vi "Yokogawa_original.vi"() -> ()   [LabVIEW 2020]
uses:
  <instrlib>/Yokogawa GX Series/Public/Data/Read Measurement Data (Analog NChan).vi
  <instrlib>/Yokogawa GX Series/Yokogawa GX Series.lvlib
panel:
  in  "prerun period":dbl=60.0
  in  "Serial Configuration":T1={"Baud Rate"=9600, "Parity"=2, "Data Bits"=8, "Flow Control"=0} {"Flow Control" items=["None", "XON/XOFF", "RTS/CTS", "XON/XOFF & RTS/CTS"]; "Data Bits" items=["7"=7, "8"=8]; "Parity" items=["None", "Odd", "Even"]; "Baud Rate" items=["1200"=1200, "2400"=2400, "4800"=4800, "9600"=9600, "19200"=19200, "38400"=38400, "57600"=57600, "115200"=115200]}
  in  "Specified\nTemperature\nLimit":dbl
  out "Time in Seconds":dbl
  out "String":string
  in  "Stop":bool
  out "Current":dbl
  out "Waveform Chart":dbl[][](graph)
  out "Current Data":dbl[](array[numeric])
  out "Unit":string[](array[string])
  out "Channel":string[](array[string])
  out "Time Stamp":timestamp
  in  "End Channel":string="0102"
  in  "Start Channel":string="0001"
  in  "VISA resource name":refnum<visa-resource-name>
  in  "Interval":dbl=5000.0
  # "Data \nacquisition \nfrequency\n(ms)"
  # "0001"
  # "0010 default \nor however many channels you want"
  # "60"
  # "Device IP On VI Max"
  # "9600"
  # "2"
  # "8"
  # "0"
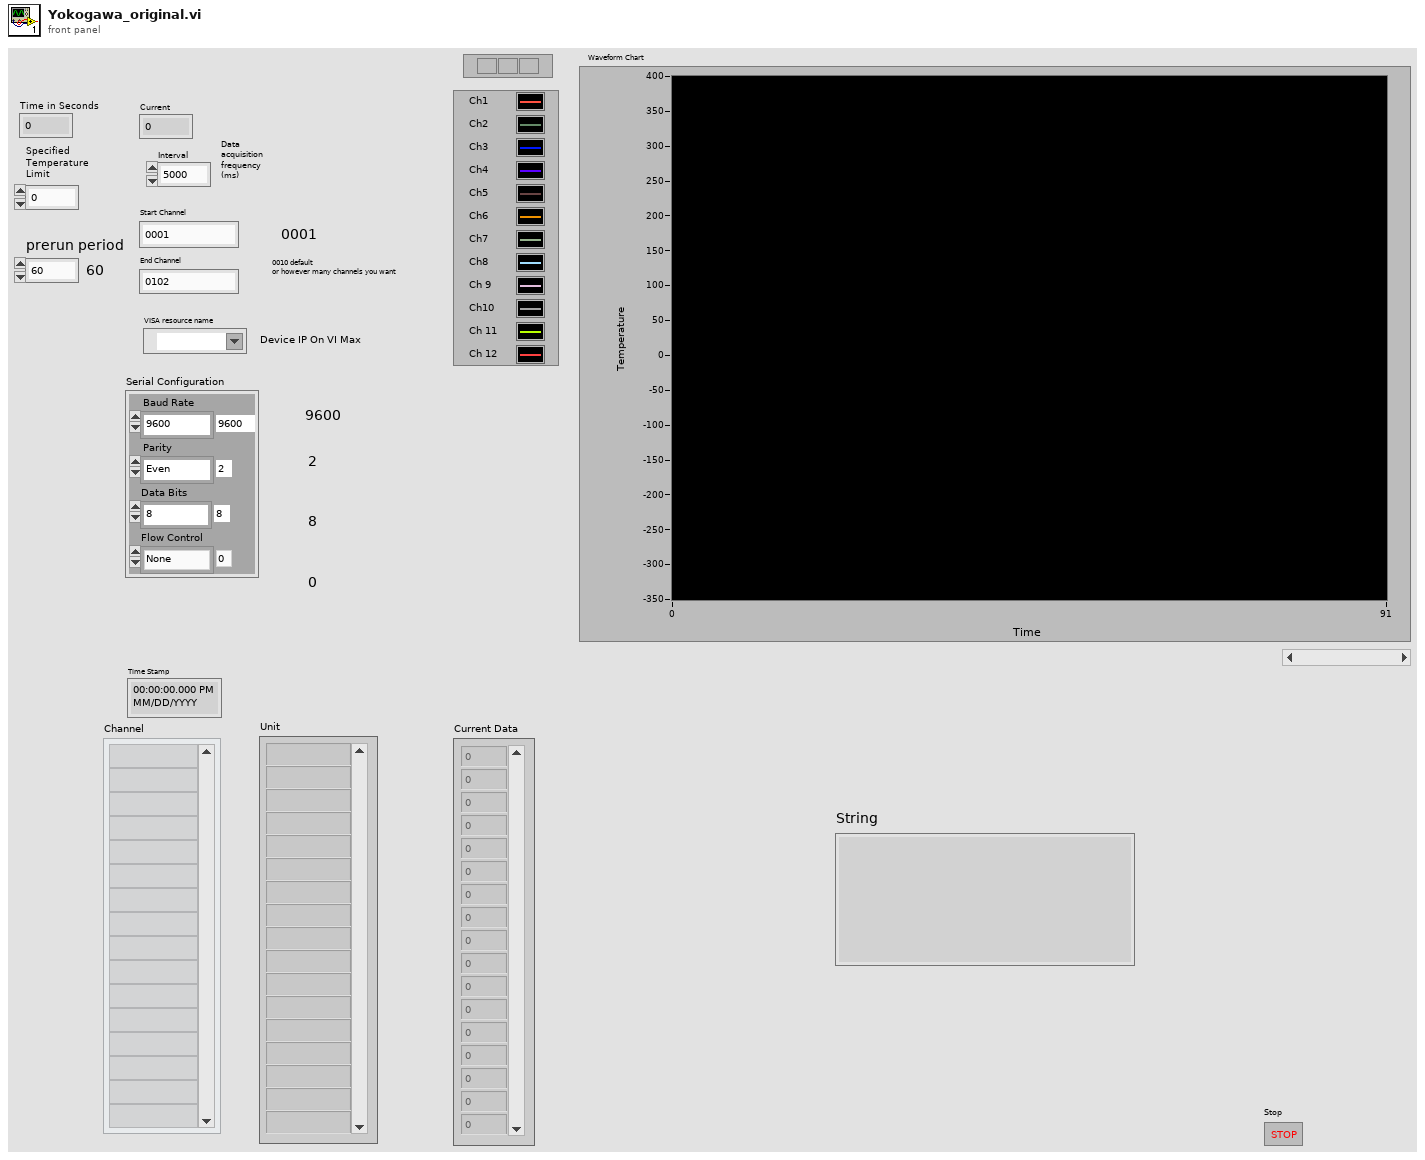
[diagram p1: front panel]
types:
  T1 = cluster{"Baud Rate":u32, "Parity":u16, "Data Bits":u16, "Flow Control":u16}
  T2 = enum16{"open", "replace", "create", "open or create", "replace or create", "replace or create with confirmation"}
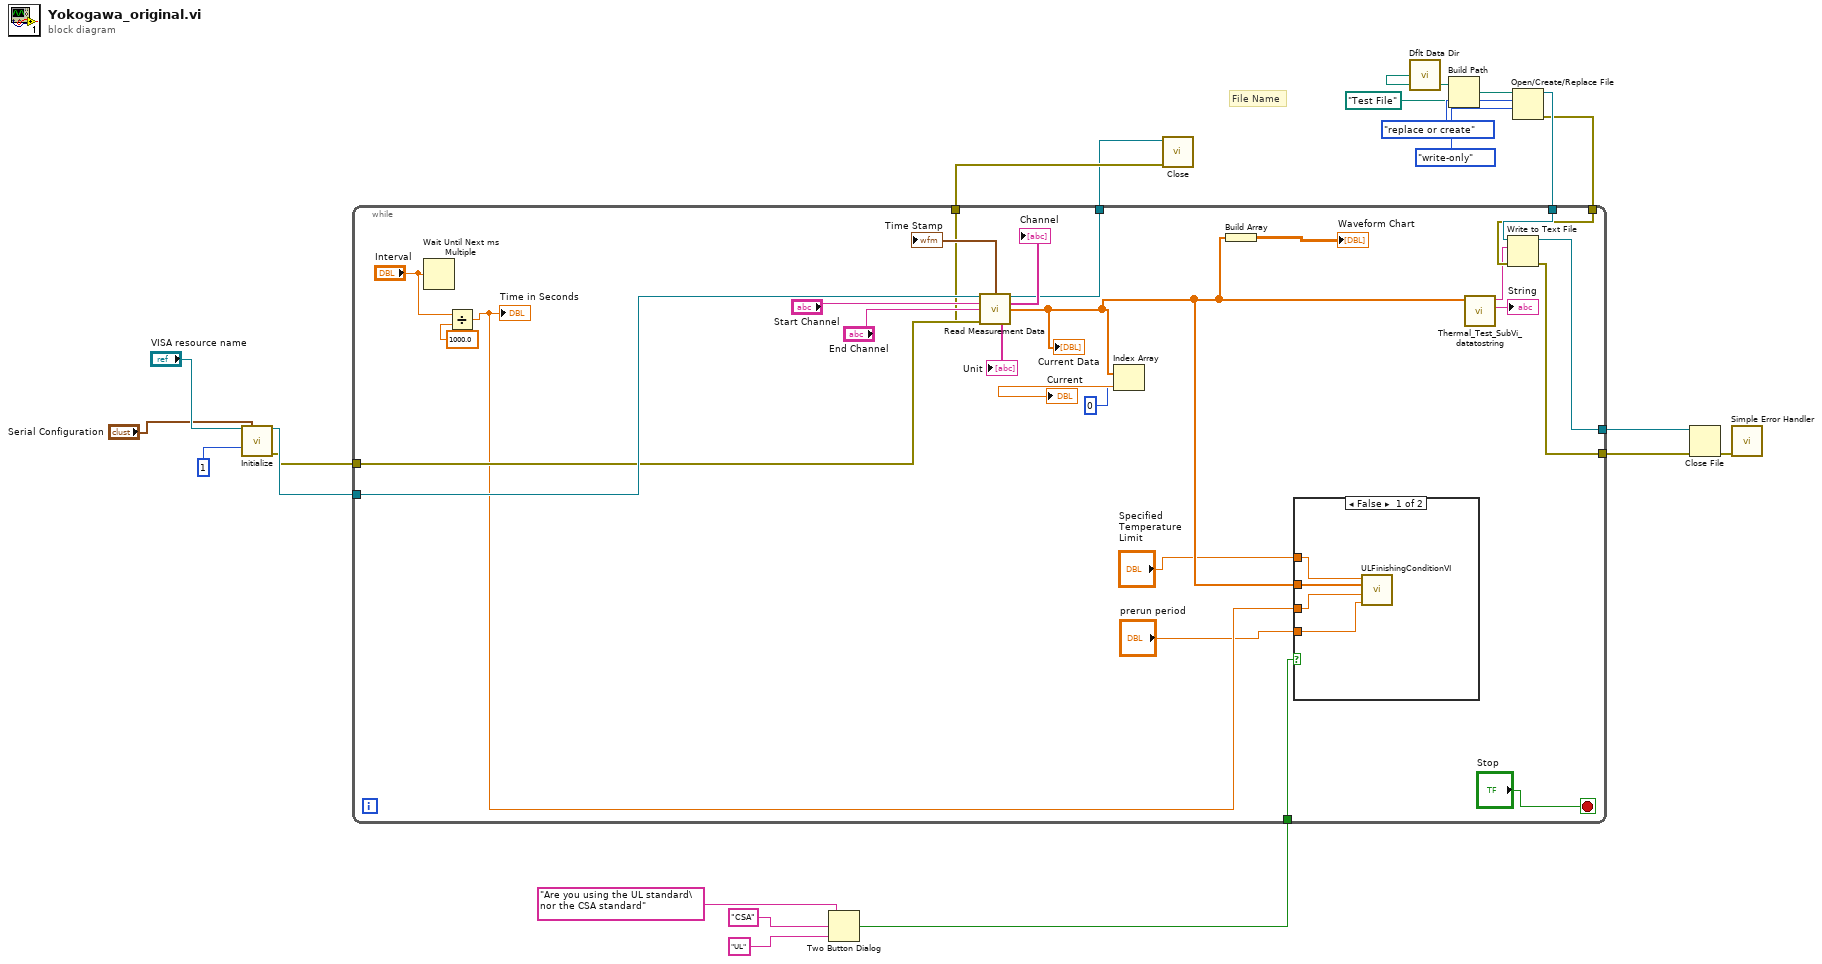
[diagram p0: block diagram]
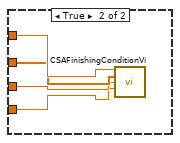
[diagram p2: hidden frame]
diagram:
  # "File Name"
  n1 = call <instrlib>:"Initialize.vi"("VISA resource name IN"="VISA resource name", "Serial Configuration"="Serial Configuration", "Serial Auth Type (0: Not Auth)"=1) -> ("VISA resource name out"=w20:refnum<visa-resource-name>, "error out"=w19:errorcluster)  [unwired: 11 in]
  n2 = Two Button Dialog(message="Are you using the UL standard\nor the CSA standard", 1:"UL", 2:"CSA") -> (T button?=w1:bool)
  n3 = call <vilib>:"Dflt Data Dir.vi"() -> ("App:Default Data Directory"=w12:path)
  n4 = Build Path(base path=w12, name or relative path=path "Test File" ("default name")) -> (appended path=w6:path)
  n5 = Open/Create/Replace File(file path (use dialog)=w6, operation (0:open)=T2."replace or create", access (0:read/write)=enum16{"read/write", "read-only", "write-only"}."write-only") -> (refnum out=w11:refnum<file>, error out=w10:errorcluster)  [unwired: 1 in, 3 out]
  n6 = while {
    tunnel: w20 -> [w41]
    tunnel: w19 -> [w40]
    tunnel: [w39] -> w17
    tunnel: [w38] -> w16
    tunnel: w11 -> [w37]
    tunnel: w10 -> [w36]
    tunnel: [w35] -> w9
    tunnel: [w34] -> w8
    tunnel: w1 -> [w22]
    stop <- "Stop" stop-if-true
    n7 = Wait Until Next ms Multiple(millisecond multiple="Interval") -> ()  [unwired: 1 out]
    n8 = Divide(x="Interval", y=1000.0) -> (x/y=w26:dbl)
    "Time in Seconds" <- w26
    n9 = call-poly <instrlib>:"Read Measurement Data.vi"("VISA resource name"=w41, "Start Channel (1)"="Start Channel", "End Channel (1)"="End Channel", "error in (no error)"=w40) -> ("Date Time"=→"Time Stamp":timestamp, "VISA resource name out"=w38:refnum<visa-resource-name>, "Channel"=→"Channel":string[], "Data"=w25:dbl[], "Unit"=→"Unit":string[], "error out"=w39:errorcluster)  [unwired: 4 in, 2 out]
    "Current Data" <- w25
    n10 = Index Array(array=w25, index=0) -> (element=→"Current":dbl)
    n11 = Build Array(w25) -> (→"Waveform Chart":dbl[][])
    n12 = case shown="False" w22 {
      tunnel: w26 -> [w49 w53]
      tunnel: w25 -> [w50 w54]
      tunnel: "Specified\nTemperature\nLimit" -> [w51 w55]
      tunnel: "prerun period" -> [w48 w52]
      frame False {
        n13 = call "ULFinishingConditionVI.vi"("prerun period"=w48, "Time in s"=w49, "Input Data"=w50, "Specified \nTemperature\nLimit\nInput"=w51) -> ()  [unwired: 8 in]
      }
      frame True {
        n14 = call "CSAFinishingConditionVi.vi"("Specified \nTemperature\nLimit\nInput"=w55, "Input Data"=w54, "Time in s"=w53, "prerun period"=w52) -> ()  [unwired: 12 in]
      }
    }
    n15 = call "Thermal_Test_SubVi_datatostring.vi"("Data"=w25) -> ("String"=→"String":string, "String 3"=w33:string)  [unwired: 9 in]
    n16 = Write to Text File(file (use dialog)=w37, text=w33, error in=w36) -> (refnum out=w35:refnum<file>, error out=w34:errorcluster)  [unwired: 1 in, 1 out]
  }
  n17 = call <instrlib>:"Close.vi"("error in (no error)"=w17, "VISA resource name"=w16) -> ()  [unwired: 9 in, 1 out]
  n18 = Close File(refnum=w9, error in=w8) -> (error out=w7:errorcluster)  [unwired: 1 out]
  n19 = call <vilib>:"Simple Error Handler.vi"("error in (no error)"=w7) -> ()  [unwired: 1 in, 8 out]
